vi "HP 3325B Function Gen.vi"(0 "marker":ext=5000000.0 format="%.3f", 1 "stop":ext=10000000.0 format="%.3f", 2 "start":ext=1000000.0 format="%.3f", 3 "sweep function (none:0)":u16(ring) items=["no sweep", "linear single", "linear cont.", "log single", "log cont."], 4 "phase (deg)":ext format="%.2f", 5 "GPIB address":i32, 6 "sweep time (S)":ext=1.0 format="%.2f", 7 "modulation (off:0)":u16(ring) items=["off", "phase", "amplitude", "amp & phase"], 8 "frequency (Hz)":ext=1000.0 format="%.3f", 9 "offset (V)":ext format="%.2f", 10 "amplitude (V)":ext=1.0 format="%.4f", 11 "signal type (dc:0)":u16(ring) items=["dc ", "sine", "square", "triangle", "pos. ramp", "neg. ramp"]) -> ()   [LabVIEW 2018]
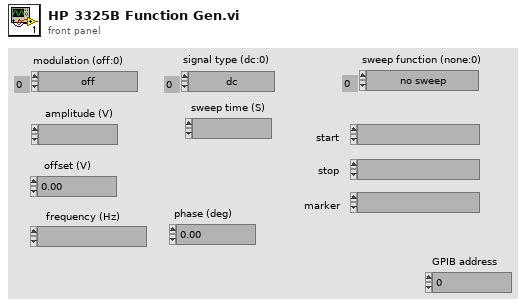
[diagram p1: front panel]
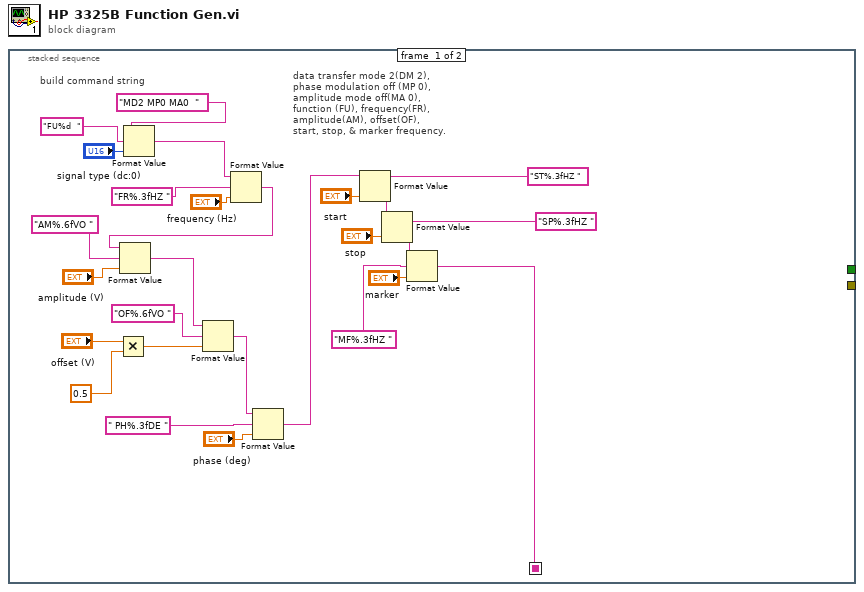
[diagram p0: block diagram]
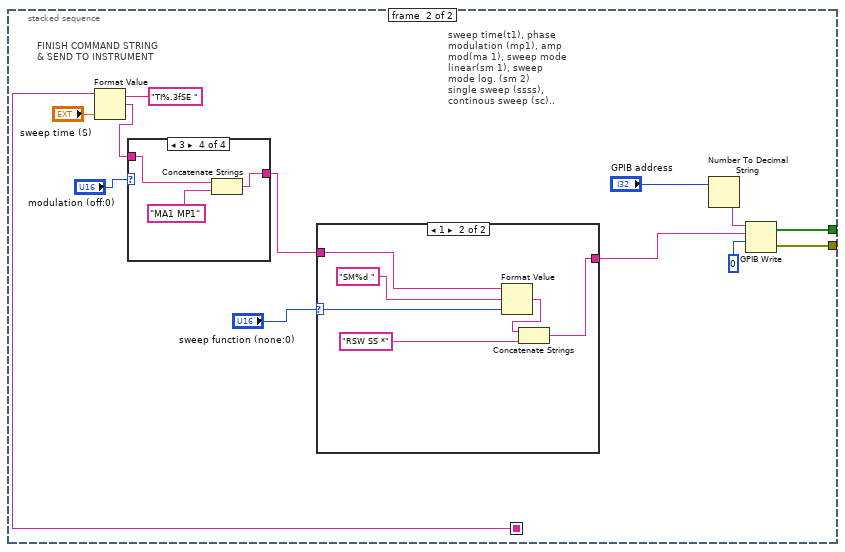
[diagram p2: hidden frame]
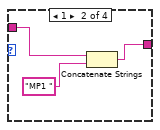
[diagram p4: hidden frame]
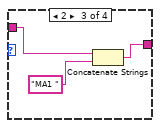
[diagram p5: hidden frame]
diagram:
  n1 = stacked-sequence {
    seq-local: [w27 _] -> [_ w39]
    tunnel: [_ w36] -> _
    tunnel: [_ w35] -> _
    frame #0 {
      # "data transfer mode 2(DM 2),\nphase modulation off (MP 0),\namplitude mode off(MA 0),\nfunction (FU), frequency(FR),\namplitude(AM), offset(OF),\nstart, stop, & marker frequency."
      # "build command string"
      n2 = Multiply(x="offset (V)", y=0.5) -> (x*y=w4:ext)
      n3 = Format Value(string ("")="MD2 MP0 MA0  ", format string="FU%d  ", value (0)="signal type (dc:0)") -> (output string=w10:string)
      n4 = Format Value(string ("")=w10, format string="FR%.3fHZ ", value (0)="frequency (Hz)") -> (output string=w13:string)
      n5 = Format Value(string ("")=w13, format string="AM%.6fVO ", value (0)="amplitude (V)") -> (output string=w15:string)
      n6 = Format Value(string ("")=w15, format string="OF%.6fVO ", value (0)=w4) -> (output string=w7:string)
      n7 = Format Value(string ("")=w7, format string=" PH%.3fDE ", value (0)="phase (deg)") -> (output string=w6:string)
      n8 = Format Value(string ("")=w6, format string="ST%.3fHZ ", value (0)="start") -> (output string=w20:string)
      n9 = Format Value(string ("")=w20, format string="SP%.3fHZ ", value (0)="stop") -> (output string=w24:string)
      n10 = Format Value(string ("")=w24, format string="MF%.3fHZ ", value (0)="marker") -> (output string=w27:string)
    }
    frame #1 {
      # "sweep time(t1), phase\nmodulation (mp1), amp\nmod(ma 1), sweep mode\nlinear(sm 1), sweep \nmode log. (sm 2)\nsingle sweep (ssss),\ncontinous sweep (sc).."
      # "FINISH COMMAND STRING\n& SEND TO INSTRUMENT"
      n11 = Format Value(string ("")=w39, format string="TI%.3fSE ", value (0)="sweep time (S)") -> (output string=w29:string)
      n12 = case shown="3" "modulation (off:0)" {
        tunnel: w29 -> [w41 w44 w46 w49]
        tunnel: [w41 w42 w45 w48] -> w28
        frame 0, Default {
        }
        frame 1 {
          n13 = Concatenate Strings(w44, "MP1 ") -> (w42:string)
        }
        frame 2 {
          n14 = Concatenate Strings(w46, "MA1 ") -> (w45:string)
        }
        frame 3 {
          n15 = Concatenate Strings(w49, "MA1 MP1") -> (w48:string)
        }
      }
      n16 = case shown="1" "sweep function (none:0)" {
        selector: "sweep function (none:0)" -> [_ w55]
        tunnel: w28 -> [w51 w57]
        tunnel: [w51 w53] -> w32
        frame 0, Default {
        }
        frame 1 {
          n17 = Format Value(string ("")=w57, format string="SM%d ", value (0)=w55) -> (output string=w54:string)
          n18 = Concatenate Strings(w54, "RSW SS *") -> (w53:string)
        }
      }
      n19 = Number To Decimal String(number="GPIB address") -> (decimal integer string=w33:string)  [unwired: 1 in]
      n20 = GPIB Write(0:w33, 1:w32, 2:0) -> (5:w36:bool[], 6:w35:errorcluster)  [unwired: 1 in, 1 out]
    }
  }
